vi "MotionMagicTorqueCurrentFOC SetControl.vi"(0 "DeviceReference":T1, 1 "StopSendingOtherRequests":bool=TRUE, 2 "Position":dbl, 3 "FeedForward":dbl, 4 "Slot":i32, 5 "OverrideCoastDurNeutral":bool, 6 "LimitForwardMotion":bool, 7 "error in":errorcluster, 8 "LimitReverseMotion":bool, 9 "IgnoreHardwareLimits":bool, 10 "UseTimesync":bool, 18 "Update Frequency (Hz)":dbl=100.0) -> (20 "DeviceReference Out":T1, 27 "error out":errorcluster)   [LabVIEW 2023]
doc: "Requests Motion Magic® to target a final position using a motion profile. Users can optionally provide a torque current feedforward.\nMotion Magic® produces a motion profile in real-time while attempting to honor the Cruise Velocity, Acceleration, and (optional) Jerk specified via the Motion Magic® configuration values. This control mode does not use the Expo_kV or Expo_kA configs.\nTarget position can be changed on-the-fly and Motion Magic® will do its best to adjust the profile. This control mode is based on torque current, so relevant closed-loop gains will use Amperes for the numerator."
uses:
  Users/test.DESKTOP-CORY/Documents/PhoenixProLabVIEWGeneration/CopyDown/DeviceReference.ctl
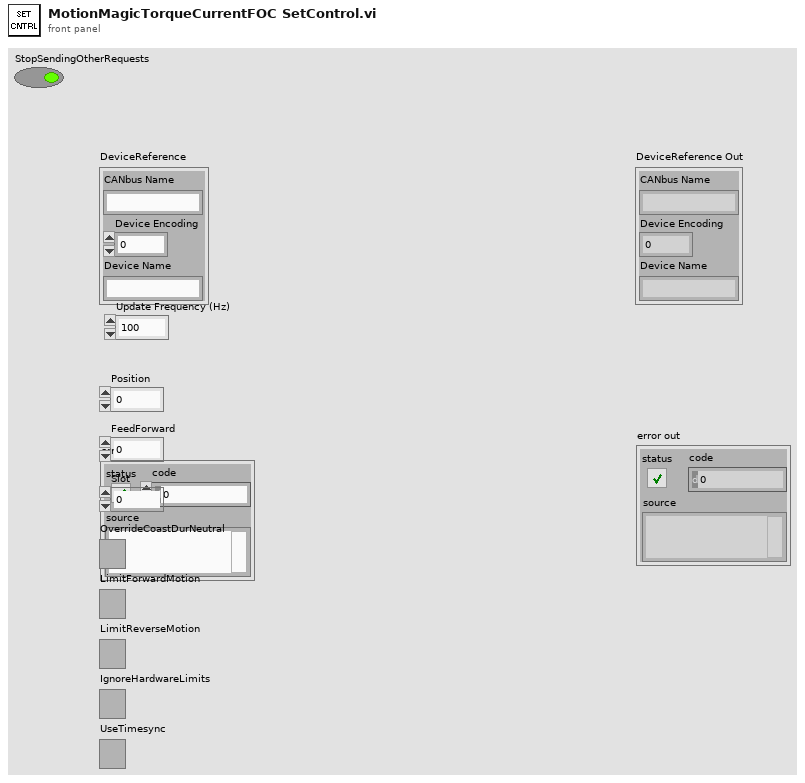
[diagram p1: front panel]
types:
  T1 = typedef "DeviceReference.ctl" = cluster{"CANbus Name":string, "Device Encoding":u32, "Device Name":string}
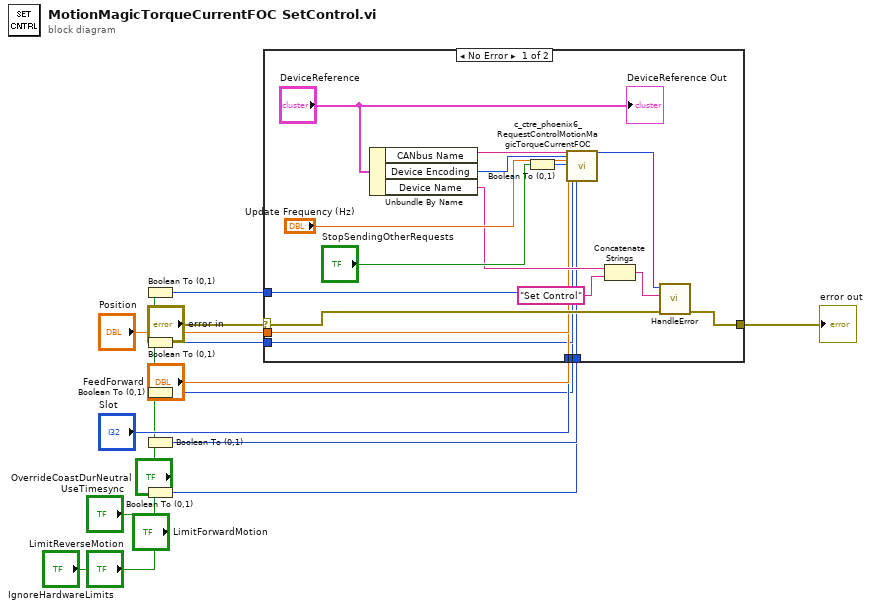
[diagram p0: block diagram]
diagram:
  n1 = Boolean To (0,1)(Boolean="OverrideCoastDurNeutral") -> (0, 1=w9:i16)
  n2 = Boolean To (0,1)(Boolean="LimitForwardMotion") -> (0, 1=w7:i16)
  n3 = Boolean To (0,1)(Boolean="LimitReverseMotion") -> (0, 1=w5:i16)
  n4 = Boolean To (0,1)(Boolean="IgnoreHardwareLimits") -> (0, 1=w3:i16)
  n5 = Boolean To (0,1)(Boolean="UseTimesync") -> (0, 1=w1:i16)
  n6 = case shown="No Error" "error in" {
    selector: "error in" -> [w28 w36]
    tunnel: [w27 w36] -> w14
    tunnel: "Position" -> [w23 _]
    tunnel: "FeedForward" -> [w22 _]
    tunnel: "Slot" -> [w21 _]
    tunnel: w9 -> [w20 _]
    tunnel: w7 -> [w19 _]
    tunnel: w5 -> [w18 _]
    tunnel: w3 -> [w17 _]
    tunnel: w1 -> [w16 _]
    frame No Error {
      n7 = Unbundle By Name("DeviceReference") -> ("CANbus Name"=w34:string, "Device Encoding"=w33:u32, "Device Name"=w26:string)
      n8 = Boolean To (0,1)(Boolean="StopSendingOtherRequests") -> (0, 1=w30:i16)
      n9 = call <vilib>:"c_ctre_phoenix6_RequestControlMotionMagicTorqueCurrentFOC.vi"("String 2"=w34, "Numeric 2"=w33, "Numeric 3"="Update Frequency (Hz)", "Numeric 4"=w30, "Numeric 5"=w23, "Numeric 6"=w22, "Numeric 7"=w21, "Numeric 8"=w20, "Numeric 9"=w19, "Numeric 10"=w18, "Numeric 11"=w17, 11:w16) -> ("Numeric"=w29:i32)  [unwired: 14 in, 1 out]
      n10 = Concatenate Strings(w26, "Set Control" ("origin")) -> (w24:string)
      n11 = call "HandleError.vi"("error in"=w28, "origin"=w24, "Status"=w29) -> ("error out"=w27:errorcluster)  [unwired: 8 in]
      "DeviceReference Out" <- "DeviceReference"
    }
    frame Error {
    }
  }
  "error out" <- w14
